vi "Update robot location and direction.vi"(0 "Map input":dbl[][](array[numeric]), 1 "Actual robot location":dbl[](array[numeric]), 2 "Robot angle":dbl) -> (7 "Map Output":dbl[][](array[numeric]), 8 "Centre location":dbl[](array[numeric]))   [LabVIEW 2015]
panel:
  out "Robot Direction":string
  out "Robot Location":dbl[](array[numeric])
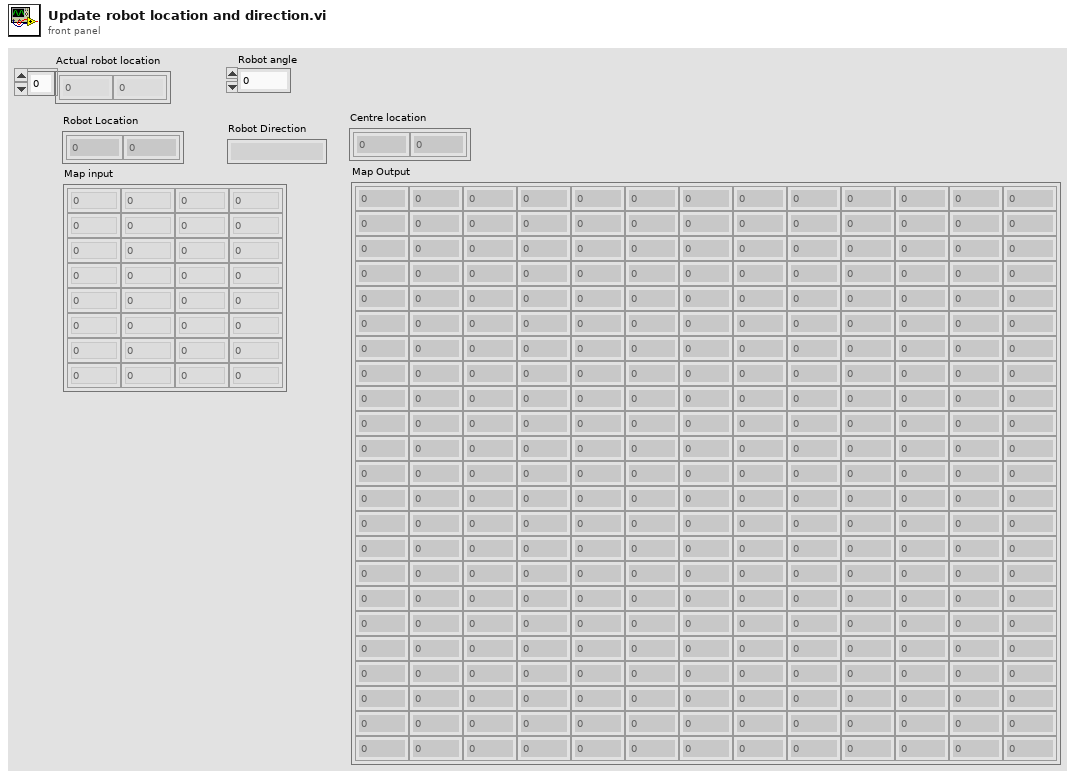
[diagram p1: front panel]
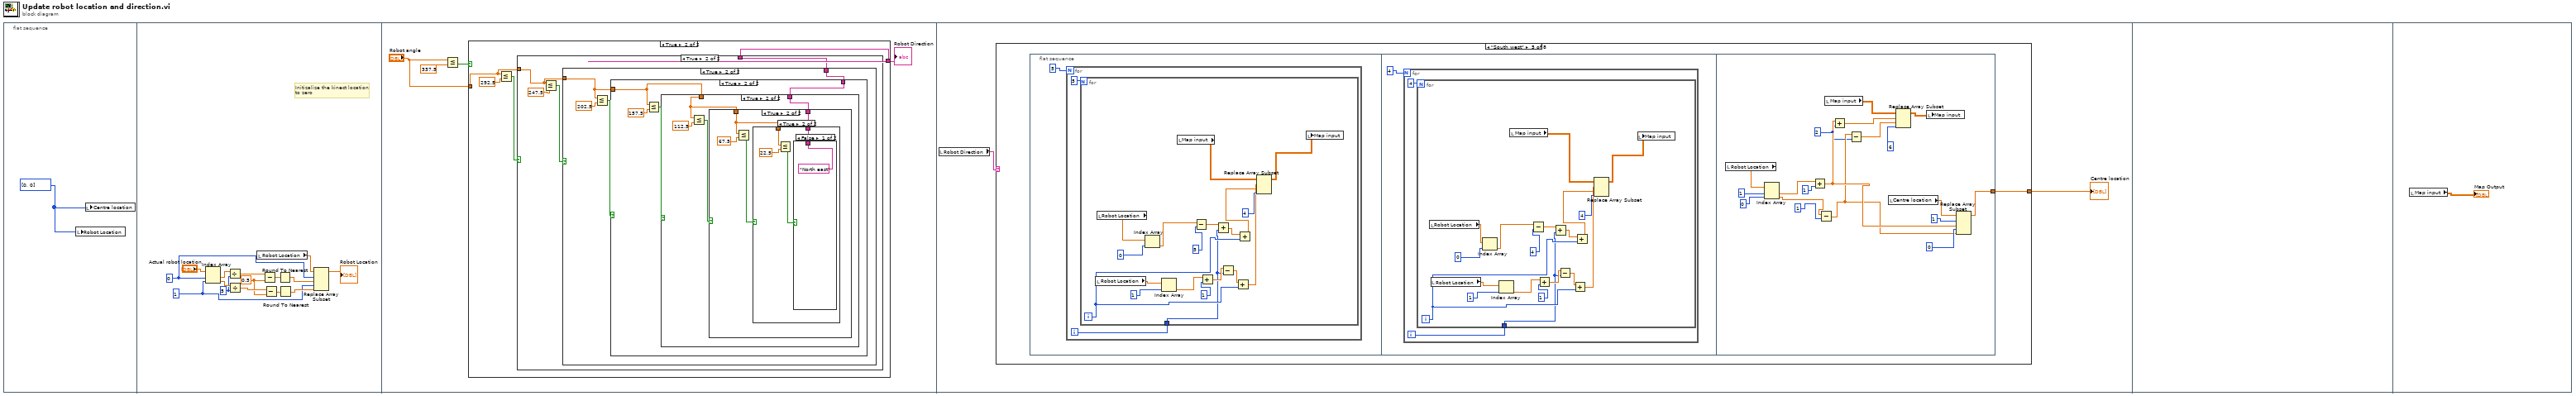
[diagram p0: block diagram]
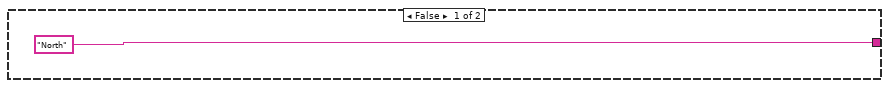
[diagram p2: hidden frame]
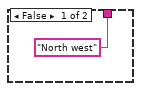
[diagram p3: hidden frame]
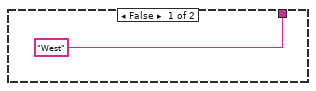
[diagram p4: hidden frame]
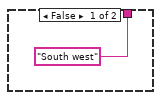
[diagram p5: hidden frame]
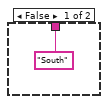
[diagram p6: hidden frame]
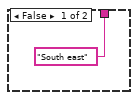
[diagram p7: hidden frame]
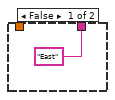
[diagram p8: hidden frame]
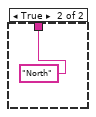
[diagram p9: hidden frame]
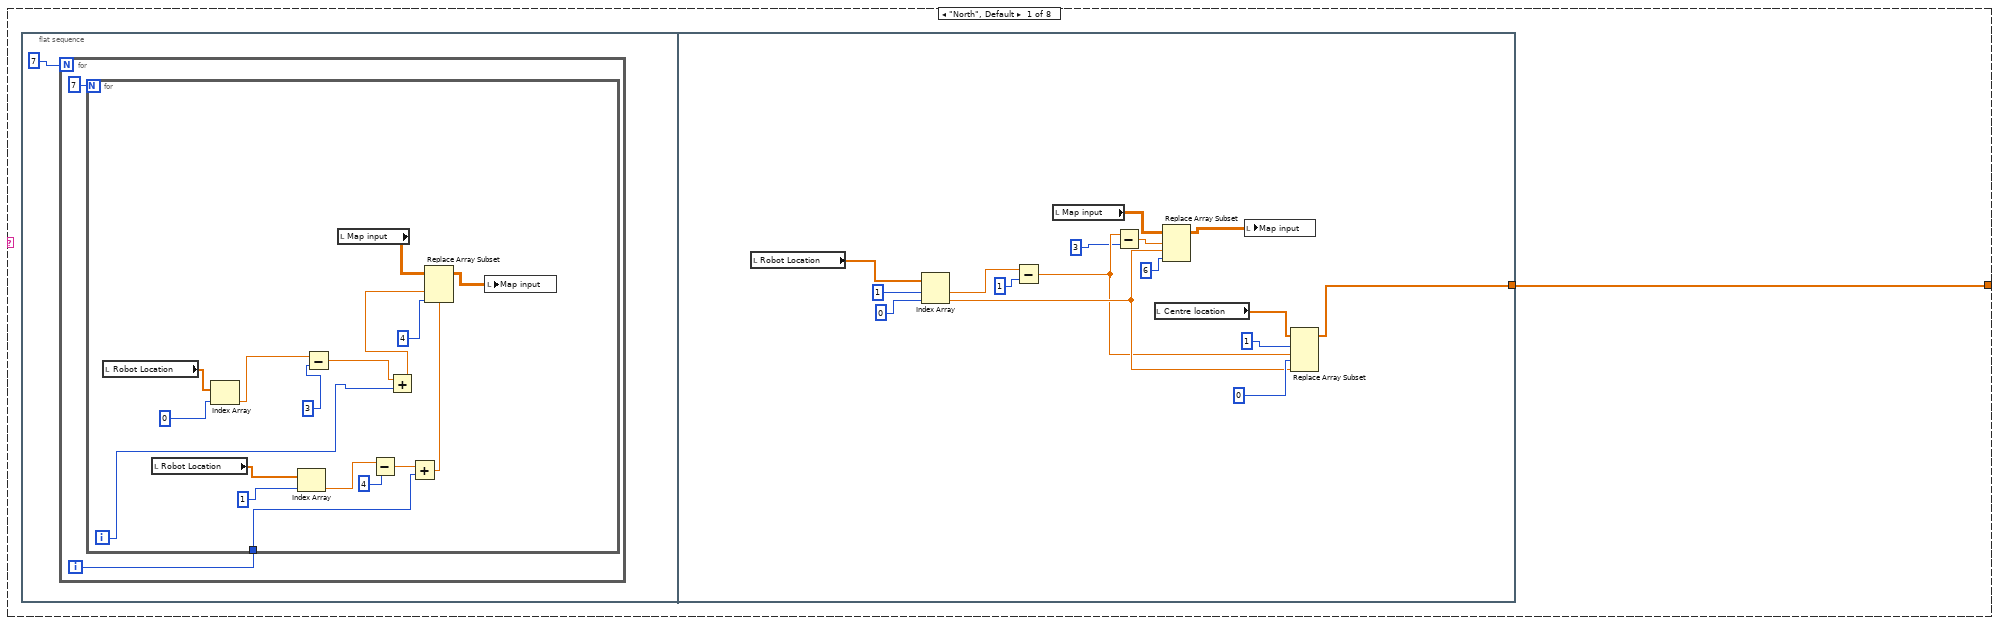
[diagram p10: hidden frame]
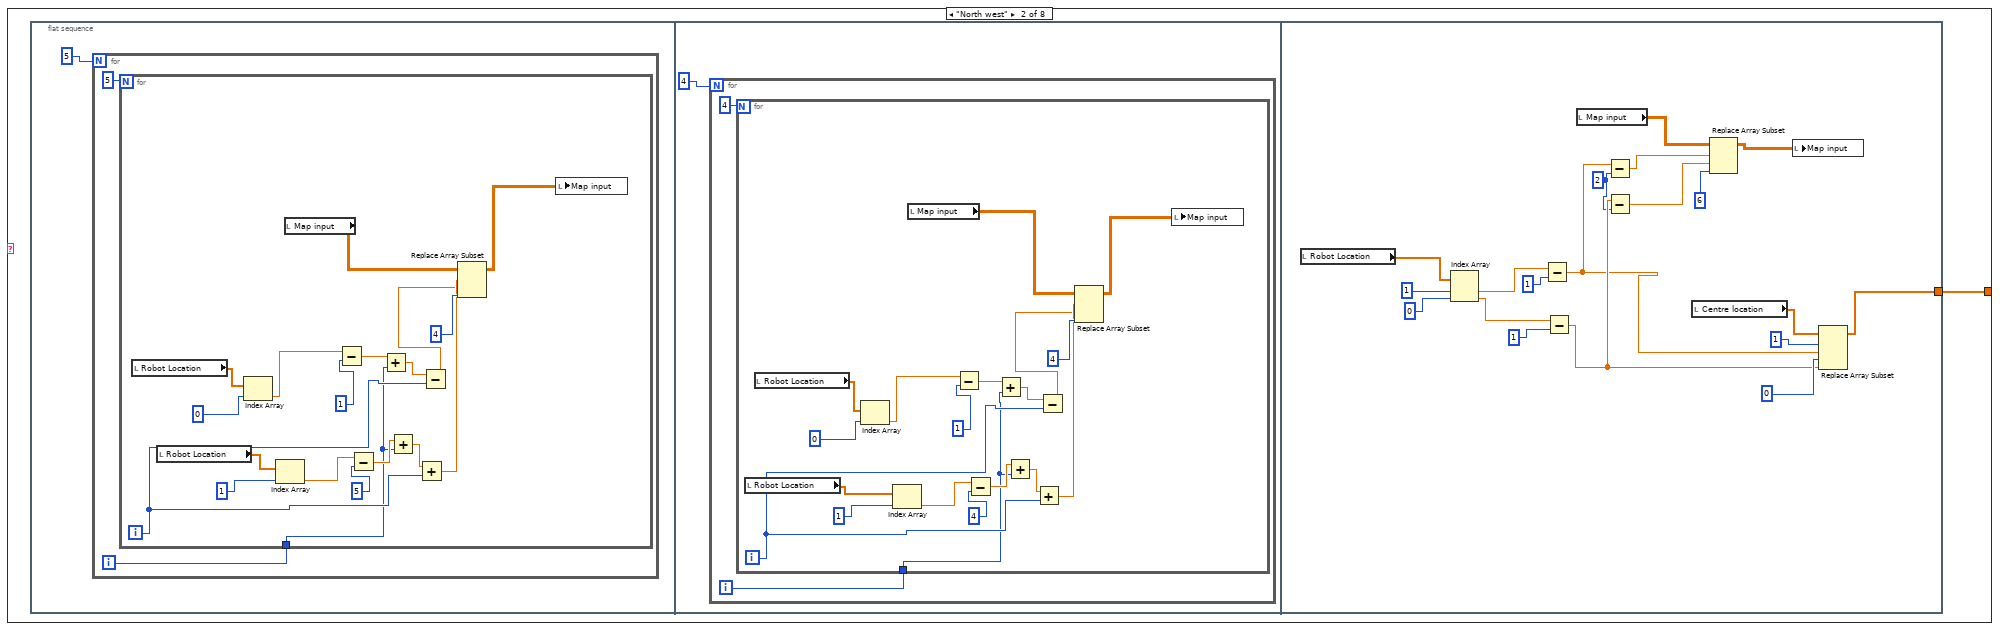
[diagram p11: hidden frame]
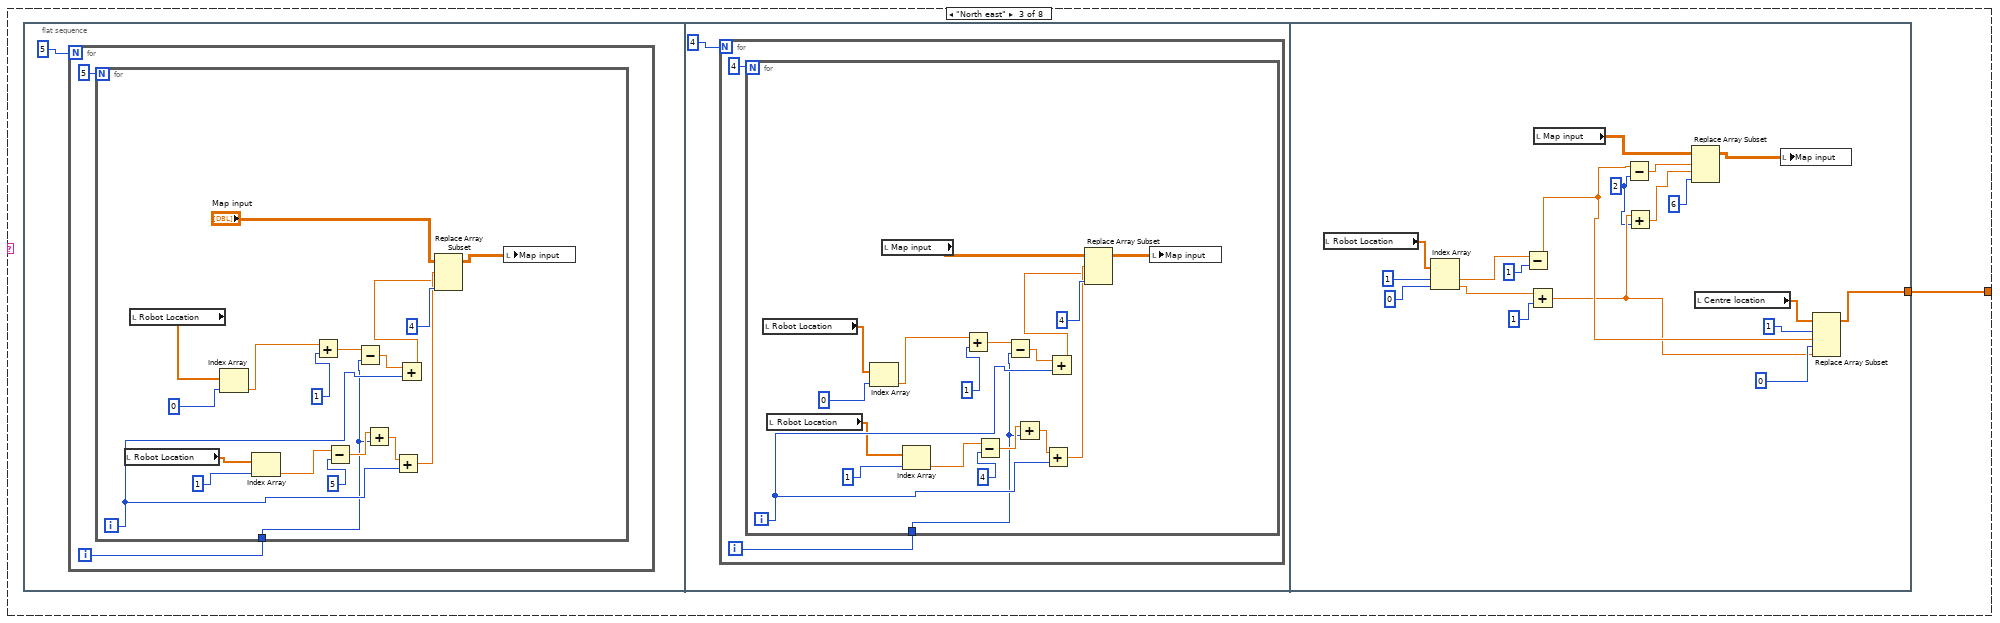
[diagram p12: hidden frame]
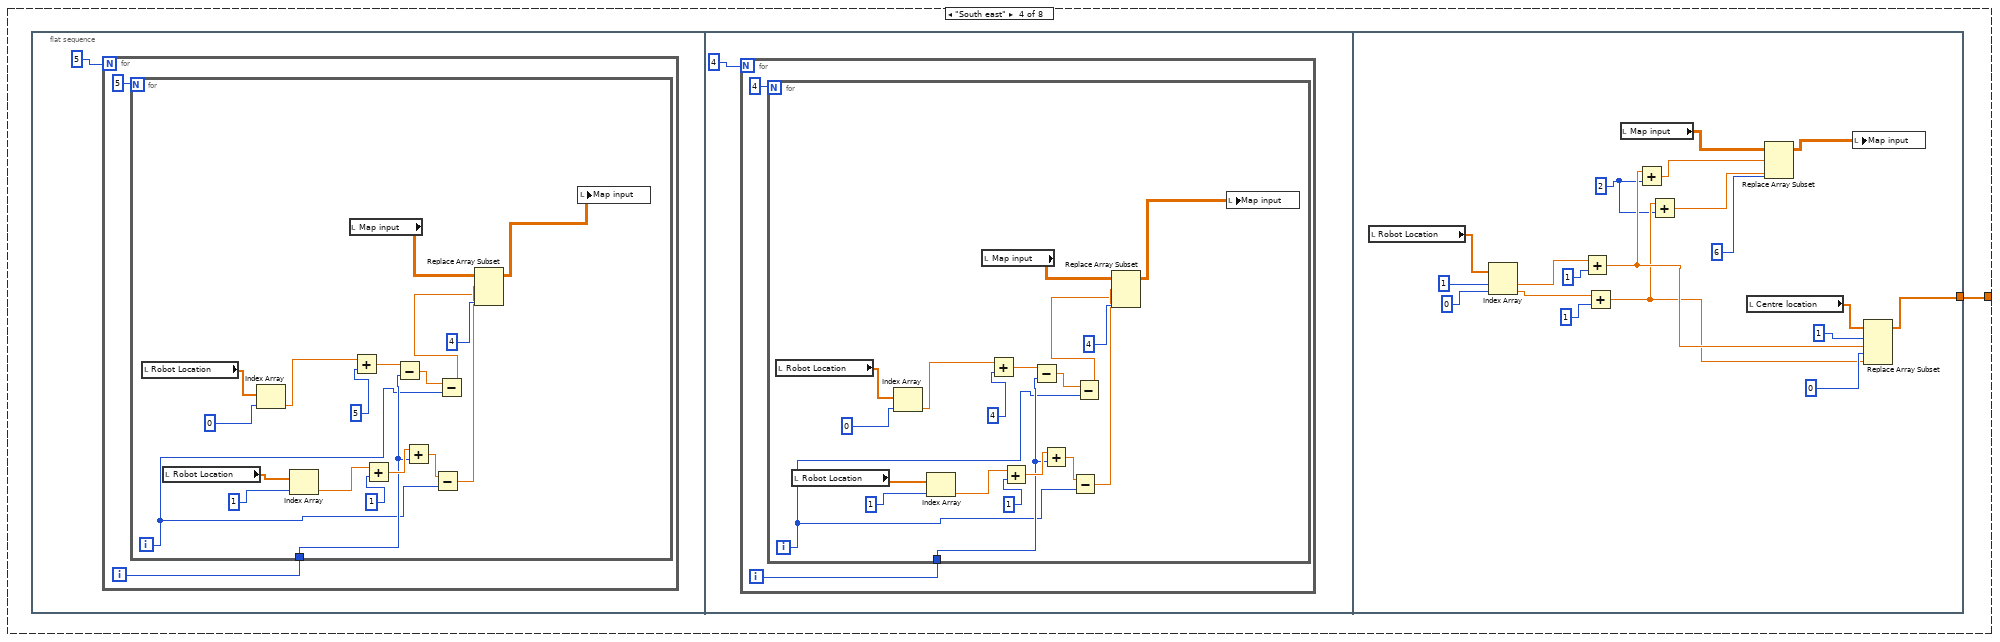
[diagram p13: hidden frame]
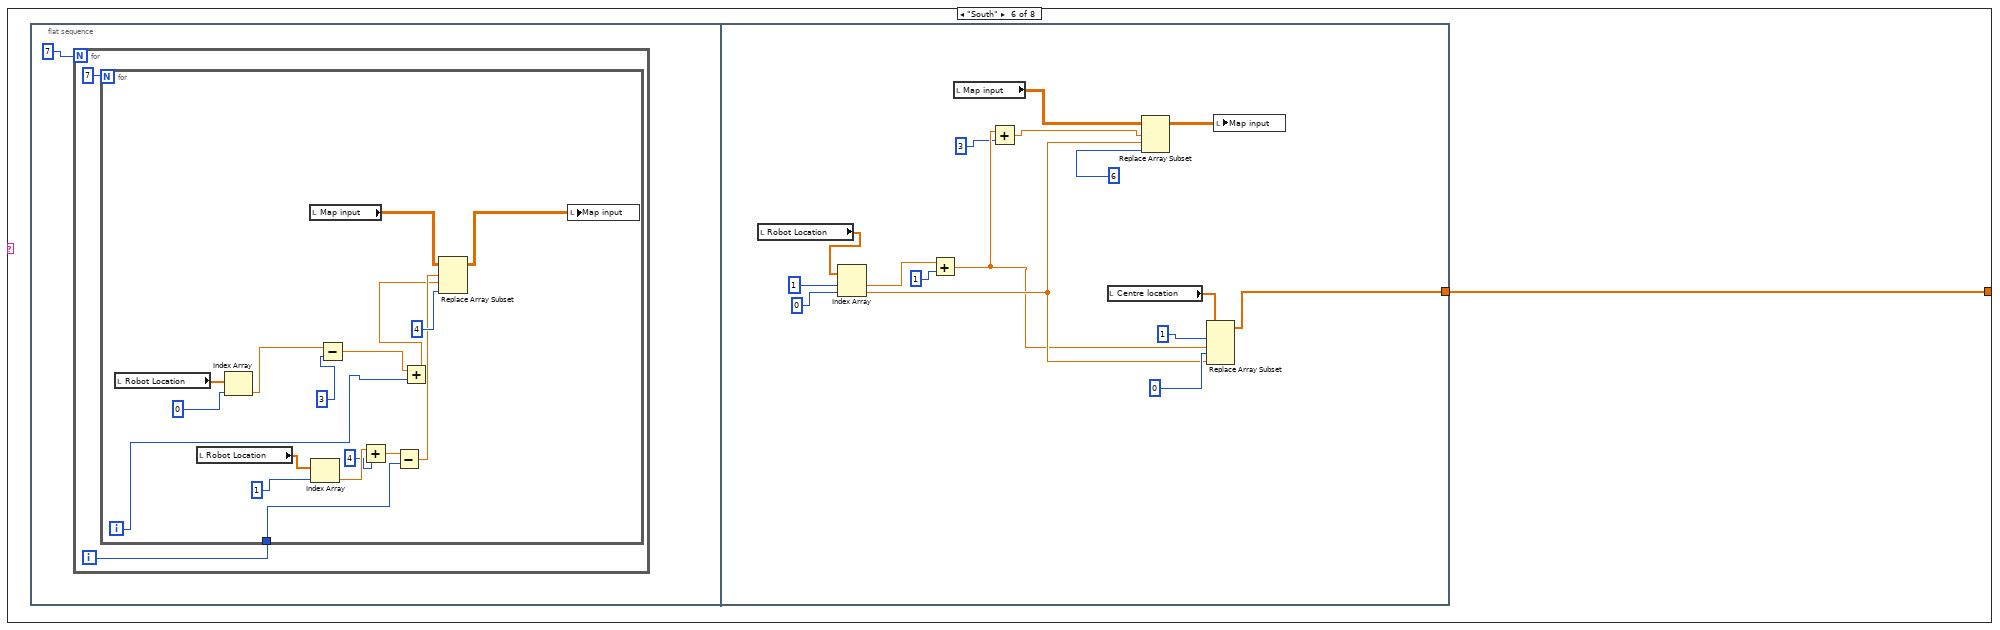
[diagram p14: hidden frame]
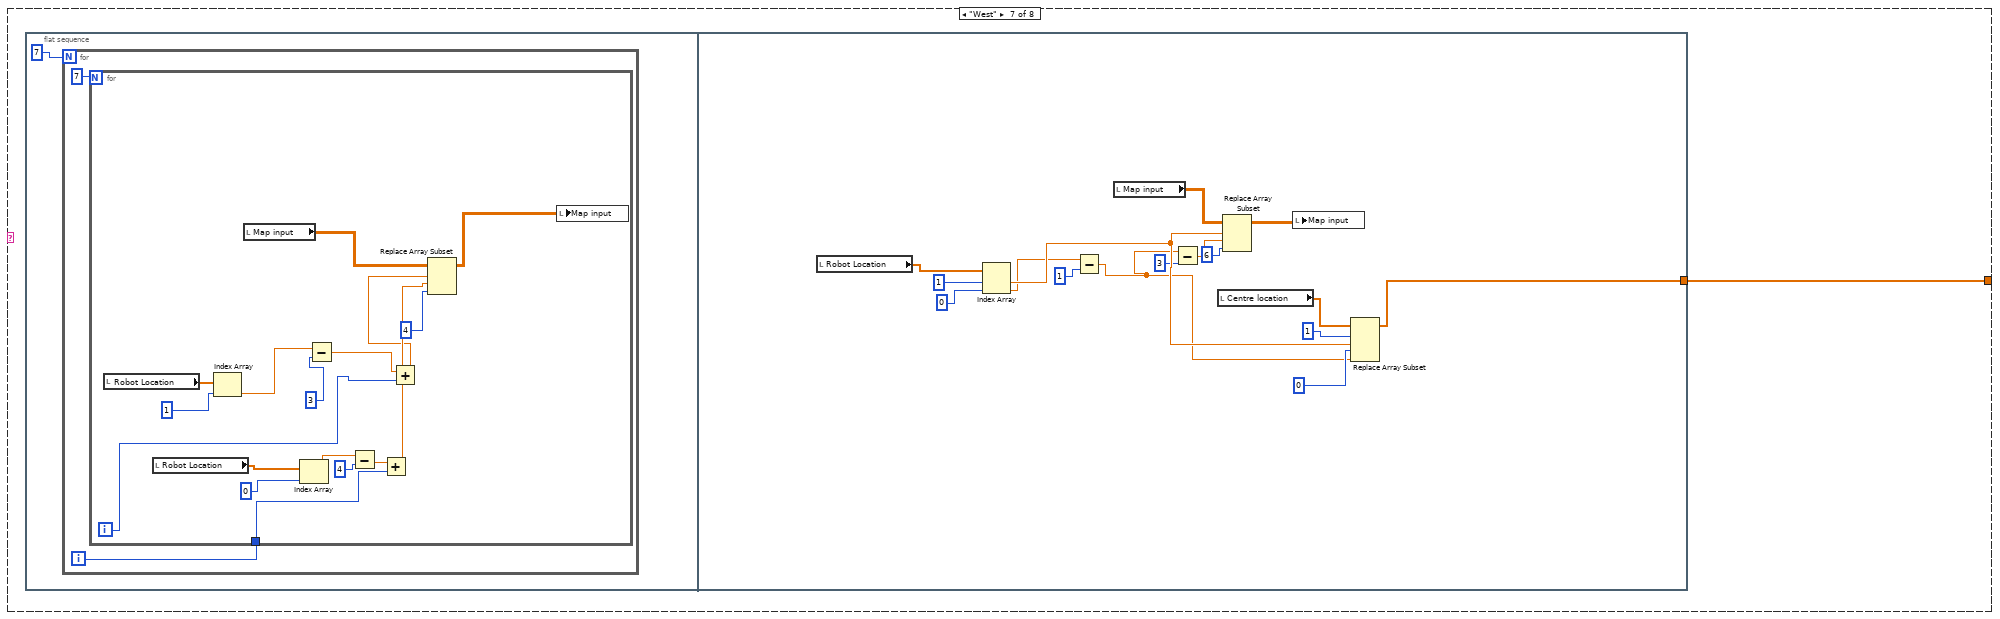
[diagram p15: hidden frame]
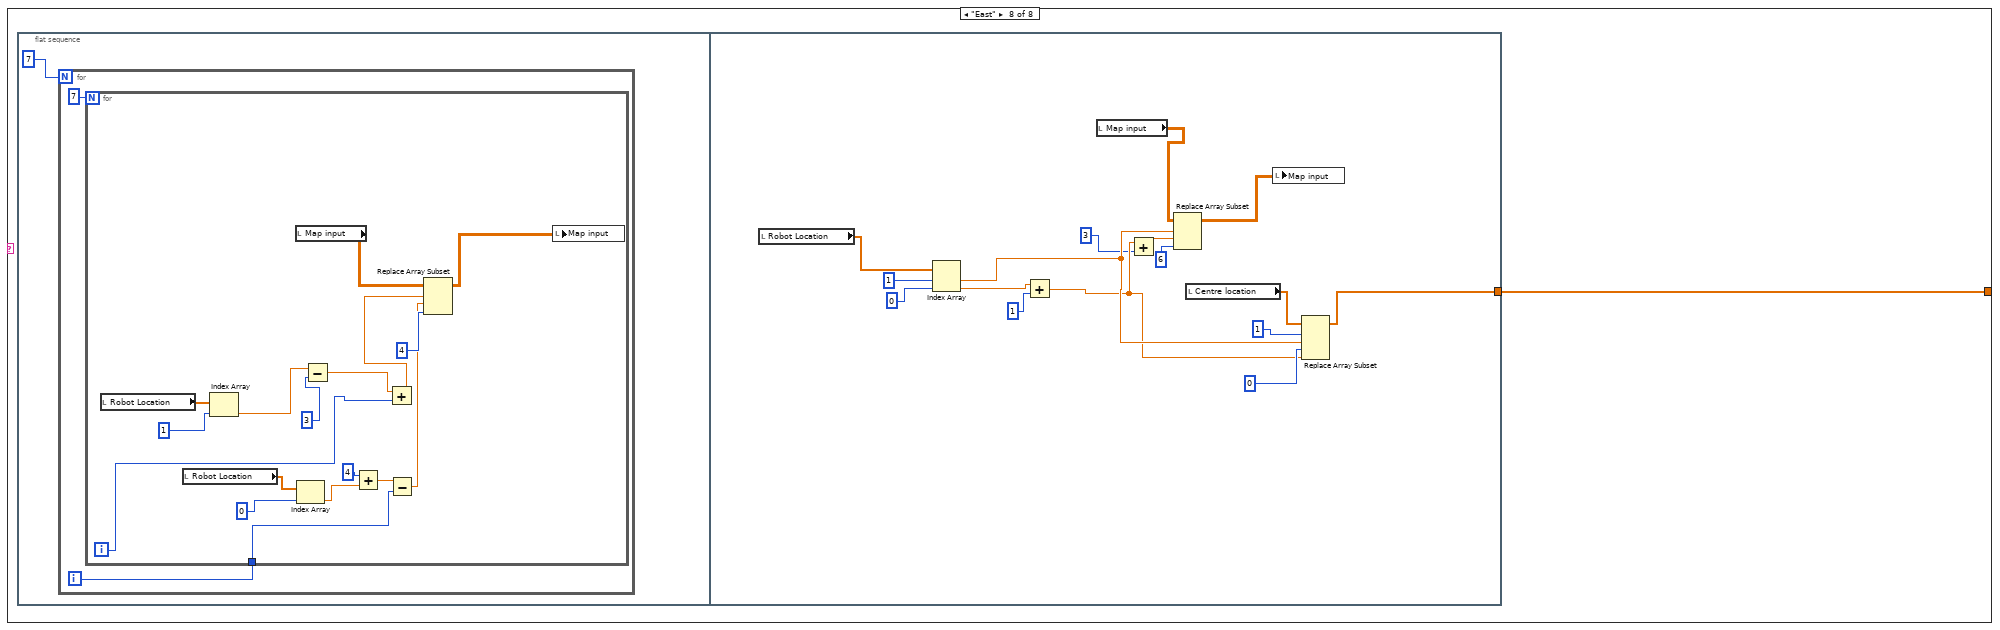
[diagram p16: hidden frame]
diagram:
  n1 = flat-sequence {
    frame #0 {
      w1 = i32[] [0, 0]
      n2 = local write "Robot Location"(w1) -> ()
      n3 = local write "Centre location"(w1) -> ()
    }
    frame #1 {
      w8 = 0.5
      w11 = 5
      w2 = 1
      w3 = 0
      # "Initizalize the kinect location \nto zero"
      n4 = Index Array(array="Actual robot location", index #1=w3, index #2=w2) -> (element #1=w13:dbl, element #2=w12:dbl)
      n5 = Divide(x=w13, y=w11) -> (x/y=w9:dbl)
      n6 = Divide(x=w12, y=w11) -> (x/y=w10:dbl)
      n7 = local read "Robot Location"() -> (w14:dbl[])
      n8 = Subtract(x=w9, y=w8) -> (x-y=w7:dbl)
      n9 = Subtract(x=w10, y=w8) -> (x-y=w6:dbl)
      n10 = Round To Nearest(number=w7) -> (nearest integer value=w5:dbl)
      n11 = Round To Nearest(number=w6) -> (nearest integer value=w4:dbl)
      n12 = Replace Array Subset(array=w14, new element #1=w5, index #1=w3, new element #2=w4, index #2=w2) -> (→"Robot Location":dbl[])
    }
    frame #2 {
      n13 = Less Or Equal?(x="Robot angle", y=337.5) -> (x <= y?=w19:bool)
      n14 = case shown="True" w19 {
        tunnel: ["North" w23] -> w20
        tunnel: "Robot angle" -> [_ w22]
        frame False {
        }
        frame True {
          n15 = Less Or Equal?(x=w22, y=292.5) -> (x <= y?=w24:bool)
          n16 = case shown="True" w24 {
            tunnel: ["North west" w28] -> w23
            tunnel: w22 -> [_ w27]
            frame False {
            }
            frame True {
              n17 = Less Or Equal?(x=w27, y=247.5) -> (x <= y?=w29:bool)
              n18 = case shown="True" w29 {
                tunnel: ["West" w33] -> w28
                tunnel: w27 -> [_ w32]
                frame False {
                }
                frame True {
                  n19 = Less Or Equal?(x=w32, y=202.5) -> (x <= y?=w34:bool)
                  n20 = case shown="True" w34 {
                    tunnel: ["South west" w38] -> w33
                    tunnel: w32 -> [_ w37]
                    frame False {
                    }
                    frame True {
                      n21 = Less Or Equal?(x=w37, y=157.5) -> (x <= y?=w39:bool)
                      n22 = case shown="True" w39 {
                        tunnel: ["South" w43] -> w38
                        tunnel: w37 -> [_ w42]
                        frame False {
                        }
                        frame True {
                          n23 = Less Or Equal?(x=w42, y=112.5) -> (x <= y?=w44:bool)
                          n24 = case shown="True" w44 {
                            tunnel: ["South east" w48] -> w43
                            tunnel: w42 -> [_ w47]
                            frame False {
                            }
                            frame True {
                              n25 = Less Or Equal?(x=w47, y=67.5) -> (x <= y?=w49:bool)
                              n26 = case shown="True" w49 {
                                tunnel: ["East" w52] -> w48
                                tunnel: w47 -> [_ w54]
                                frame False {
                                }
                                frame True {
                                n27 = Less Or Equal?(x=w54, y=22.5) -> (x <= y?=w53:bool)
                                n28 = case shown="False" w53 {
                                tunnel: ["North east" "North"] -> w52
                                frame False {
                                }
                                frame True {
                                }
                                }
                                }
                              }
                            }
                          }
                        }
                      }
                    }
                  }
                }
              }
            }
          }
        }
      }
      "Robot Direction" <- w20
    }
    frame #3 {
      n29 = local read "Robot Direction"() -> (w58:string)
      n30 = case shown="\"South west\"" w58 {
        tunnel: [w60 w97 w161 w225 w289 w353 w390 w427] -> w59
        frame "North", Default {
          n31 = flat-sequence {
            tunnel: [w90] -> w60
            frame #0 {
              n32 = for {
                N: 7 -> [_]
                i -> [w62]
                n33 = for {
                  N: 7 -> [_]
                  tunnel: w62 -> [w72]
                  i -> [w76]
                  n34 = local read "Robot Location"() -> (w68:dbl[])
                  n35 = local read "Robot Location"() -> (w67:dbl[])
                  n36 = Index Array(array=w68, index=0) -> (element=w69:dbl)
                  n37 = Index Array(array=w67, index=1) -> (element=w66:dbl)
                  n38 = Subtract(x=w69, y=3) -> (x-y=w75:dbl)
                  n39 = local read "Map input"() -> (w71:dbl[][])
                  n40 = Subtract(x=w66, y=4) -> (x-y=w65:dbl)
                  n41 = Add(x=w75, y=w76) -> (x+y=w73:dbl)
                  n42 = Add(x=w65, y=w72) -> (x+y=w74:dbl)
                  n43 = Replace Array Subset(array=w71, new element=4, index (row)=w74, index (col)=w73) -> (w70:dbl[][])
                  n44 = local write "Map input"(w70) -> ()
                }
              }
            }
            frame #1 {
              n45 = local read "Robot Location"() -> (w87:dbl[])
              n46 = Index Array(array=w87, index #1=1, index #2=0) -> (element #1=w93:dbl, element #2=w86:dbl)
              n47 = Subtract(x=w93, y=1) -> (x-y=w82:dbl)
              n48 = local read "Map input"() -> (w88:dbl[][])
              n49 = Subtract(x=w82, y=3) -> (x-y=w83:dbl)
              n50 = local read "Centre location"() -> (w84:dbl[])
              n51 = Replace Array Subset(array=w88, new element=6, index (row)=w83, index (col)=w86) -> (w89:dbl[][])
              n52 = local write "Map input"(w89) -> ()
              n53 = Replace Array Subset(array=w84, new element #1=w82, index #1=1, new element #2=w86, index #2=0) -> (w90:dbl[])
            }
          }
        }
        frame "North west" {
          n54 = flat-sequence {
            tunnel: [w151] -> w97
            frame #0 {
              n55 = for {
                N: 5 -> [_]
                i -> [w99]
                n56 = for {
                  N: 5 -> [_]
                  tunnel: w99 -> [w101]
                  i -> [w112]
                  n57 = local read "Robot Location"() -> (w107:dbl[])
                  n58 = local read "Robot Location"() -> (w106:dbl[])
                  n59 = Index Array(array=w107, index=0) -> (element=w113:dbl)
                  n60 = Index Array(array=w106, index=1) -> (element=w111:dbl)
                  n61 = local read "Map input"() -> (w105:dbl[][])
                  n62 = Subtract(x=w113, y=1) -> (x-y=w103:dbl)
                  n63 = Subtract(x=w111, y=5) -> (x-y=w109:dbl)
                  n64 = Add(x=w103, y=w101) -> (x+y=w102:dbl)
                  n65 = Add(x=w109, y=w101) -> (x+y=w108:dbl)
                  n66 = Add(x=w108, y=w112) -> (x+y=w115:dbl)
                  n67 = Subtract(x=w102, y=w112) -> (x-y=w114:dbl)
                  n68 = Replace Array Subset(array=w105, new element=4, index (row)=w115, index (col)=w114) -> (w104:dbl[][])
                  n69 = local write "Map input"(w104) -> ()
                }
              }
            }
            frame #1 {
              n70 = for {
                N: 4 -> [_]
                i -> [w121]
                n71 = for {
                  N: 4 -> [_]
                  tunnel: w121 -> [w128]
                  i -> [w134]
                  n72 = local read "Robot Location"() -> (w123:dbl[])
                  n73 = local read "Robot Location"() -> (w124:dbl[])
                  n74 = Index Array(array=w124, index=0) -> (element=w135:dbl)
                  n75 = Index Array(array=w123, index=1) -> (element=w133:dbl)
                  n76 = local read "Map input"() -> (w126:dbl[][])
                  n77 = Subtract(x=w135, y=1) -> (x-y=w131:dbl)
                  n78 = Subtract(x=w133, y=4) -> (x-y=w130:dbl)
                  n79 = Add(x=w131, y=w128) -> (x+y=w129:dbl)
                  n80 = Add(x=w130, y=w128) -> (x+y=w127:dbl)
                  n81 = Add(x=w127, y=w134) -> (x+y=w137:dbl)
                  n82 = Subtract(x=w129, y=w134) -> (x-y=w136:dbl)
                  n83 = Replace Array Subset(array=w126, new element=4, index (row)=w137, index (col)=w136) -> (w125:dbl[][])
                  n84 = local write "Map input"(w125) -> ()
                }
              }
            }
            frame #2 {
              w142 = 2
              n85 = local read "Robot Location"() -> (w150:dbl[])
              n86 = Index Array(array=w150, index #1=1, index #2=0) -> (element #1=w157:dbl, element #2=w148:dbl)
              n87 = Subtract(x=w157, y=1) -> (x-y=w145:dbl)
              n88 = Subtract(x=w148, y=1) -> (x-y=w146:dbl)
              n89 = local read "Map input"() -> (w153:dbl[][])
              n90 = Subtract(x=w145, y=w142) -> (x-y=w144:dbl)
              n91 = Subtract(x=w146, y=w142) -> (x-y=w143:dbl)
              n92 = local read "Centre location"() -> (w152:dbl[])
              n93 = Replace Array Subset(array=w153, new element=6, index (row)=w144, index (col)=w143) -> (w154:dbl[][])
              n94 = local write "Map input"(w154) -> ()
              n95 = Replace Array Subset(array=w152, new element #1=w145, index #1=1, new element #2=w146, index #2=0) -> (w151:dbl[])
            }
          }
        }
        frame "North east" {
          n96 = flat-sequence {
            tunnel: [w215] -> w161
            frame #0 {
              n97 = for {
                N: 5 -> [_]
                i -> [w163]
                n98 = for {
                  N: 5 -> [_]
                  tunnel: w163 -> [w170]
                  i -> [w176]
                  n99 = local read "Robot Location"() -> (w167:dbl[])
                  n100 = local read "Robot Location"() -> (w168:dbl[])
                  n101 = Index Array(array=w168, index=0) -> (element=w177:dbl)
                  n102 = Index Array(array=w167, index=1) -> (element=w175:dbl)
                  n103 = Add(x=w177, y=1) -> (x+y=w173:dbl)
                  n104 = Subtract(x=w175, y=5) -> (x-y=w172:dbl)
                  n105 = Subtract(x=w173, y=w170) -> (x-y=w171:dbl)
                  n106 = Add(x=w172, y=w170) -> (x+y=w169:dbl)
                  n107 = Add(x=w169, y=w176) -> (x+y=w179:dbl)
                  n108 = Add(x=w171, y=w176) -> (x+y=w178:dbl)
                  n109 = Replace Array Subset(array="Map input", new element=4, index (row)=w179, index (col)=w178) -> (w166:dbl[][])
                  n110 = local write "Map input"(w166) -> ()
                }
              }
            }
            frame #1 {
              n111 = for {
                N: 4 -> [_]
                i -> [w185]
                n112 = for {
                  N: 4 -> [_]
                  tunnel: w185 -> [w187]
                  i -> [w198]
                  n113 = local read "Robot Location"() -> (w189:dbl[])
                  n114 = local read "Robot Location"() -> (w188:dbl[])
                  n115 = Index Array(array=w189, index=0) -> (element=w199:dbl)
                  n116 = local read "Map input"() -> (w191:dbl[][])
                  n117 = Index Array(array=w188, index=1) -> (element=w197:dbl)
                  n118 = Add(x=w199, y=1) -> (x+y=w195:dbl)
                  n119 = Subtract(x=w197, y=4) -> (x-y=w194:dbl)
                  n120 = Subtract(x=w195, y=w187) -> (x-y=w193:dbl)
                  n121 = Add(x=w194, y=w187) -> (x+y=w192:dbl)
                  n122 = Add(x=w192, y=w198) -> (x+y=w201:dbl)
                  n123 = Add(x=w193, y=w198) -> (x+y=w200:dbl)
                  n124 = Replace Array Subset(array=w191, new element=4, index (row)=w201, index (col)=w200) -> (w190:dbl[][])
                  n125 = local write "Map input"(w190) -> ()
                }
              }
            }
            frame #2 {
              w206 = 2
              n126 = local read "Robot Location"() -> (w218:dbl[])
              n127 = Index Array(array=w218, index #1=1, index #2=0) -> (element #1=w221:dbl, element #2=w214:dbl)
              n128 = Subtract(x=w221, y=1) -> (x-y=w210:dbl)
              n129 = Add(x=w214, y=1) -> (x+y=w207:dbl)
              n130 = local read "Map input"() -> (w217:dbl[][])
              n131 = Subtract(x=w210, y=w206) -> (x-y=w209:dbl)
              n132 = Add(x=w207, y=w206) -> (x+y=w208:dbl)
              n133 = Replace Array Subset(array=w217, new element=6, index (row)=w209, index (col)=w208) -> (w212:dbl[][])
              n134 = local read "Centre location"() -> (w216:dbl[])
              n135 = local write "Map input"(w212) -> ()
              n136 = Replace Array Subset(array=w216, new element #1=w210, index #1=1, new element #2=w207, index #2=0) -> (w215:dbl[])
            }
          }
        }
        frame "South east" {
          n137 = flat-sequence {
            tunnel: [w277] -> w225
            frame #0 {
              n138 = for {
                N: 5 -> [_]
                i -> [w227]
                n139 = for {
                  N: 5 -> [_]
                  tunnel: w227 -> [w235]
                  i -> [w229]
                  n140 = local read "Robot Location"() -> (w231:dbl[])
                  n141 = local read "Robot Location"() -> (w230:dbl[])
                  n142 = Index Array(array=w231, index=0) -> (element=w241:dbl)
                  n143 = Index Array(array=w230, index=1) -> (element=w240:dbl)
                  n144 = local read "Map input"() -> (w232:dbl[][])
                  n145 = Add(x=w241, y=5) -> (x+y=w238:dbl)
                  n146 = Add(x=w240, y=1) -> (x+y=w237:dbl)
                  n147 = Subtract(x=w238, y=w235) -> (x-y=w236:dbl)
                  n148 = Add(x=w237, y=w235) -> (x+y=w234:dbl)
                  n149 = Subtract(x=w234, y=w229) -> (x-y=w243:dbl)
                  n150 = Subtract(x=w236, y=w229) -> (x-y=w242:dbl)
                  n151 = Replace Array Subset(array=w232, new element=4, index (row)=w243, index (col)=w242) -> (w233:dbl[][])
                  n152 = local write "Map input"(w233) -> ()
                }
              }
            }
            frame #1 {
              n153 = for {
                N: 4 -> [_]
                i -> [w249]
                n154 = for {
                  N: 4 -> [_]
                  tunnel: w249 -> [w257]
                  i -> [w254]
                  n155 = local read "Robot Location"() -> (w255:dbl[])
                  n156 = local read "Robot Location"() -> (w253:dbl[])
                  n157 = Index Array(array=w255, index=0) -> (element=w263:dbl)
                  n158 = Index Array(array=w253, index=1) -> (element=w262:dbl)
                  n159 = local read "Map input"() -> (w252:dbl[][])
                  n160 = Add(x=w263, y=4) -> (x+y=w260:dbl)
                  n161 = Add(x=w262, y=1) -> (x+y=w259:dbl)
                  n162 = Subtract(x=w260, y=w257) -> (x-y=w258:dbl)
                  n163 = Add(x=w259, y=w257) -> (x+y=w256:dbl)
                  n164 = Subtract(x=w256, y=w254) -> (x-y=w265:dbl)
                  n165 = Subtract(x=w258, y=w254) -> (x-y=w264:dbl)
                  n166 = Replace Array Subset(array=w252, new element=4, index (row)=w265, index (col)=w264) -> (w251:dbl[][])
                  n167 = local write "Map input"(w251) -> ()
                }
              }
            }
            frame #2 {
              w270 = 2
              n168 = local read "Robot Location"() -> (w279:dbl[])
              n169 = Index Array(array=w279, index #1=1, index #2=0) -> (element #1=w285:dbl, element #2=w276:dbl)
              n170 = Add(x=w285, y=1) -> (x+y=w274:dbl)
              n171 = Add(x=w276, y=1) -> (x+y=w271:dbl)
              n172 = local read "Map input"() -> (w281:dbl[][])
              n173 = Add(x=w274, y=w270) -> (x+y=w273:dbl)
              n174 = Add(x=w271, y=w270) -> (x+y=w272:dbl)
              n175 = local read "Centre location"() -> (w278:dbl[])
              n176 = Replace Array Subset(array=w281, new element=6, index (row)=w273, index (col)=w272) -> (w282:dbl[][])
              n177 = local write "Map input"(w282) -> ()
              n178 = Replace Array Subset(array=w278, new element #1=w274, index #1=1, new element #2=w271, index #2=0) -> (w277:dbl[])
            }
          }
        }
        frame "South west" {
          n179 = flat-sequence {
            tunnel: [w346] -> w289
            frame #0 {
              n180 = for {
                N: 5 -> [_]
                i -> [w291]
                n181 = for {
                  N: 5 -> [_]
                  tunnel: w291 -> [w299]
                  i -> [w305]
                  n182 = local read "Robot Location"() -> (w294:dbl[])
                  n183 = local read "Robot Location"() -> (w295:dbl[])
                  n184 = Index Array(array=w295, index=0) -> (element=w293:dbl)
                  n185 = Index Array(array=w294, index=1) -> (element=w304:dbl)
                  n186 = local read "Map input"() -> (w296:dbl[][])
                  n187 = Subtract(x=w293, y=5) -> (x-y=w302:dbl)
                  n188 = Add(x=w304, y=1) -> (x+y=w301:dbl)
                  n189 = Add(x=w302, y=w299) -> (x+y=w300:dbl)
                  n190 = Subtract(x=w301, y=w299) -> (x-y=w298:dbl)
                  n191 = Add(x=w298, y=w305) -> (x+y=w307:dbl)
                  n192 = Add(x=w300, y=w305) -> (x+y=w306:dbl)
                  n193 = Replace Array Subset(array=w296, new element=4, index (row)=w307, index (col)=w306) -> (w297:dbl[][])
                  n194 = local write "Map input"(w297) -> ()
                }
              }
            }
            frame #1 {
              n195 = for {
                N: 4 -> [_]
                i -> [w313]
                n196 = for {
                  N: 4 -> [_]
                  tunnel: w313 -> [w320]
                  i -> [w326]
                  n197 = local read "Robot Location"() -> (w316:dbl[])
                  n198 = local read "Robot Location"() -> (w315:dbl[])
                  n199 = Index Array(array=w316, index=0) -> (element=w327:dbl)
                  n200 = Index Array(array=w315, index=1) -> (element=w325:dbl)
                  n201 = local read "Map input"() -> (w318:dbl[][])
                  n202 = Subtract(x=w327, y=4) -> (x-y=w323:dbl)
                  n203 = Add(x=w325, y=1) -> (x+y=w322:dbl)
                  n204 = Add(x=w323, y=w320) -> (x+y=w321:dbl)
                  n205 = Subtract(x=w322, y=w320) -> (x-y=w319:dbl)
                  n206 = Add(x=w319, y=w326) -> (x+y=w329:dbl)
                  n207 = Add(x=w321, y=w326) -> (x+y=w328:dbl)
                  n208 = Replace Array Subset(array=w318, new element=4, index (row)=w329, index (col)=w328) -> (w317:dbl[][])
                  n209 = local write "Map input"(w317) -> ()
                }
              }
            }
            frame #2 {
              w334 = 2
              n210 = local read "Robot Location"() -> (w344:dbl[])
              n211 = Index Array(array=w344, index #1=1, index #2=0) -> (element #1=w349:dbl, element #2=w340:dbl)
              n212 = Add(x=w349, y=1) -> (x+y=w338:dbl)
              n213 = Subtract(x=w340, y=1) -> (x-y=w337:dbl)
              n214 = local read "Map input"() -> (w342:dbl[][])
              n215 = Add(x=w338, y=w334) -> (x+y=w335:dbl)
              n216 = Subtract(x=w337, y=w334) -> (x-y=w336:dbl)
              n217 = local read "Centre location"() -> (w345:dbl[])
              n218 = Replace Array Subset(array=w342, new element=6, index (row)=w335, index (col)=w336) -> (w343:dbl[][])
              n219 = local write "Map input"(w343) -> ()
              n220 = Replace Array Subset(array=w345, new element #1=w338, index #1=1, new element #2=w337, index #2=0) -> (w346:dbl[])
            }
          }
        }
        frame "South" {
          n221 = flat-sequence {
            tunnel: [w378] -> w353
            frame #0 {
              n222 = for {
                N: 7 -> [_]
                i -> [w355]
                n223 = for {
                  N: 7 -> [_]
                  tunnel: w355 -> [w365]
                  i -> [w369]
                  n224 = local read "Robot Location"() -> (w362:dbl[])
                  n225 = local read "Robot Location"() -> (w361:dbl[])
                  n226 = Index Array(array=w362, index=0) -> (element=w360:dbl)
                  n227 = local read "Map input"() -> (w364:dbl[][])
                  n228 = Index Array(array=w361, index=1) -> (element=w358:dbl)
                  n229 = Subtract(x=w360, y=3) -> (x-y=w368:dbl)
                  n230 = Add(x=w358, y=4) -> (x+y=w359:dbl)
                  n231 = Subtract(x=w359, y=w365) -> (x-y=w367:dbl)
                  n232 = Add(x=w368, y=w369) -> (x+y=w366:dbl)
                  n233 = Replace Array Subset(array=w364, new element=4, index (row)=w367, index (col)=w366) -> (w363:dbl[][])
                  n234 = local write "Map input"(w363) -> ()
                }
              }
            }
            frame #1 {
              n235 = local read "Robot Location"() -> (w380:dbl[])
              n236 = Index Array(array=w380, index #1=1, index #2=0) -> (element #1=w386:dbl, element #2=w379:dbl)
              n237 = Add(x=w386, y=1) -> (x+y=w376:dbl)
              n238 = local read "Map input"() -> (w381:dbl[][])
              n239 = Add(x=w376, y=3) -> (x+y=w375:dbl)
              n240 = local read "Centre location"() -> (w377:dbl[])
              n241 = Replace Array Subset(array=w381, new element=6, index (row)=w375, index (col)=w379) -> (w382:dbl[][])
              n242 = Replace Array Subset(array=w377, new element #1=w376, index #1=1, new element #2=w379, index #2=0) -> (w378:dbl[])
              n243 = local write "Map input"(w382) -> ()
            }
          }
        }
        frame "West" {
          n244 = flat-sequence {
            tunnel: [w419] -> w390
            frame #0 {
              n245 = for {
                N: 7 -> [_]
                i -> [w392]
                n246 = for {
                  N: 7 -> [_]
                  tunnel: w392 -> [w404]
                  i -> [w406]
                  n247 = local read "Robot Location"() -> (w399:dbl[])
                  n248 = local read "Robot Location"() -> (w398:dbl[])
                  n249 = Index Array(array=w399, index=1) -> (element=w397:dbl)
                  n250 = local read "Map input"() -> (w401:dbl[][])
                  n251 = Index Array(array=w398, index=0) -> (element=w394:dbl)
                  n252 = Subtract(x=w397, y=3) -> (x-y=w405:dbl)
                  n253 = Subtract(x=w394, y=4) -> (x-y=w396:dbl)
                  n254 = Add(x=w396, y=w404) -> (x+y=w403:dbl)
                  n255 = Add(x=w405, y=w406) -> (x+y=w402:dbl)
                  n256 = Replace Array Subset(array=w401, new element=4, index (row)=w402, index (col)=w403) -> (w400:dbl[][])
                  n257 = local write "Map input"(w400) -> ()
                }
              }
            }
            frame #1 {
              n258 = local read "Robot Location"() -> (w426:dbl[])
              n259 = Index Array(array=w426, index #1=1, index #2=0) -> (element #1=w415:dbl, element #2=w414:dbl)
              n260 = Subtract(x=w414, y=1) -> (x-y=w412:dbl)
              n261 = local read "Map input"() -> (w417:dbl[][])
              n262 = Subtract(x=w412, y=3) -> (x-y=w413:dbl)
              n263 = local read "Centre location"() -> (w420:dbl[])
              n264 = Replace Array Subset(array=w417, new element=6, index (row)=w415, index (col)=w413) -> (w418:dbl[][])
              n265 = local write "Map input"(w418) -> ()
              n266 = Replace Array Subset(array=w420, new element #1=w415, index #1=1, new element #2=w412, index #2=0) -> (w419:dbl[])
            }
          }
        }
        frame "East" {
          n267 = flat-sequence {
            tunnel: [w458] -> w427
            frame #0 {
              n268 = for {
                N: 7 -> [_]
                i -> [w429]
                n269 = for {
                  N: 7 -> [_]
                  tunnel: w429 -> [w436]
                  i -> [w438]
                  n270 = local read "Robot Location"() -> (w444:dbl[])
                  n271 = local read "Robot Location"() -> (w442:dbl[])
                  n272 = Index Array(array=w444, index=1) -> (element=w440:dbl)
                  n273 = local read "Map input"() -> (w447:dbl[][])
                  n274 = Index Array(array=w442, index=0) -> (element=w432:dbl)
                  n275 = Subtract(x=w440, y=3) -> (x-y=w437:dbl)
                  n276 = Add(x=4, y=w432) -> (x+y=w433:dbl)
                  n277 = Add(x=w437, y=w438) -> (x+y=w434:dbl)
                  n278 = Subtract(x=w433, y=w436) -> (x-y=w435:dbl)
                  n279 = Replace Array Subset(array=w447, new element=4, index (row)=w434, index (col)=w435) -> (w446:dbl[][])
                  n280 = local write "Map input"(w446) -> ()
                }
              }
            }
            frame #1 {
              n281 = local read "Robot Location"() -> (w455:dbl[])
              n282 = Index Array(array=w455, index #1=1, index #2=0) -> (element #1=w451:dbl, element #2=w452:dbl)
              n283 = Add(x=w452, y=1) -> (x+y=w449:dbl)
              n284 = local read "Map input"() -> (w456:dbl[][])
              n285 = Add(x=w449, y=3) -> (x+y=w450:dbl)
              n286 = Replace Array Subset(array=w456, new element=6, index (row)=w451, index (col)=w450) -> (w457:dbl[][])
              n287 = local read "Centre location"() -> (w453:dbl[])
              n288 = local write "Map input"(w457) -> ()
              n289 = Replace Array Subset(array=w453, new element #1=w451, index #1=1, new element #2=w449, index #2=0) -> (w458:dbl[])
            }
          }
        }
      }
      "Centre location" <- w59
    }
    frame #4 {
    }
    frame #5 {
      n290 = local read "Map input"() -> (→"Map Output":dbl[][])
    }
  }
